vi "Self Configure.vi"(8 "error in":errorcluster, 11 "MLTFNC in":refnum<class "MLTFNC.lvclass">) -> (0 "error out":errorcluster, 3 "MLTFNC out":refnum<class "MLTFNC.lvclass">)   [LabVIEW 2019, in "MLTFNC.lvlib" / "MLTFNC.lvclass"]
doc: "Children of Instruments must override this routine and call the parent method. \nThis routine is implemented to allow each instrument to read its specific configuration keys and implement any default configuration settings.\n\nThis routine already calls Connect and Self Test Routines."
uses:
  Library/MLTFNC.lvclass
  builds/Instruments/Instruments.lvlibp/Library/Instruments.lvclass
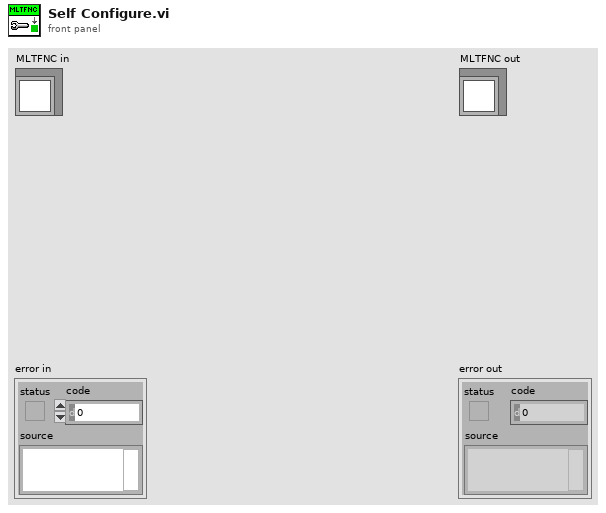
[diagram p1: front panel]
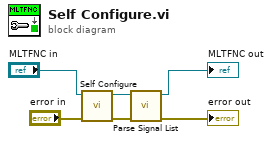
[diagram p0: block diagram]
diagram:
  n1 = call-parent "Self Configure.vi"("error in"="error in", "Instruments in"="MLTFNC in") -> ("error out"=w3:errorcluster, "Instruments out"=w4:refnum<class "MLTFNC.lvclass">)  [unwired: 8 in]
  n2 = call "Parse Signal List.vi"("error in"=w3, "MLTFNC in"=w4) -> ("error out"=→"error out":errorcluster, "MLTFNC out"=→"MLTFNC out":refnum<class "MLTFNC.lvclass">)  [unwired: 8 in]
